vi "Count_Coincidences.vi"(0 "Time-Current":dbl, 1 "Coincidence Window":dbl, 5 "Reverse?":bool, 9 "Time - Previous":dbl, 11 "Expected Delay":dbl, 13 "Coincidences In":u32) -> (4 "Delay":dbl, 6 "Is Coincidence?":bool, 10 "Coincidences Out":u32, 15 "Shifted Delay":dbl)   [LabVIEW 2023]
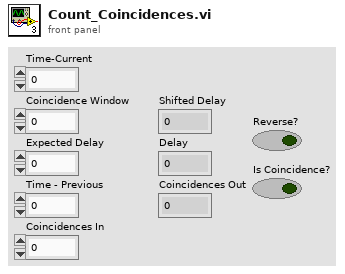
[diagram p1: front panel]
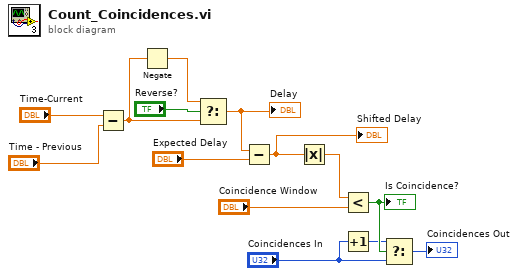
[diagram p0: block diagram]
diagram:
  n1 = Subtract(x="Time-Current", y="Time - Previous") -> (x-y=w2:dbl)
  n2 = Negate(x=w2) -> (-x=w3:dbl)
  n3 = Select(t=w3, s="Reverse?", f=w2) -> (s? t:f=w5:dbl)
  "Delay" <- w5
  n4 = Subtract(x=w5, y="Expected Delay") -> (x-y=w1:dbl)
  "Shifted Delay" <- w1
  n5 = Absolute Value(x=w1) -> (abs(x)=w9:dbl)
  n6 = Less?(x=w9, y="Coincidence Window") -> (x < y?=w14:bool)
  "Is Coincidence?" <- w14
  n7 = Increment(x="Coincidences In") -> (x+1=w12:u32)
  n8 = Select(t=w12, s=w14, f="Coincidences In") -> (s? t:f=→"Coincidences Out":u32)
